vi "Fire Logging.vi"(11 "error in":errorcluster) -> ()   [LabVIEW 2015]
doc: "Converts an array of data to a row of tab-separated columns, prepends the timestamp column, and terminates each row with the end of line character."
uses:
  <vilib>/Rock Robotics/Network Tables/NT Read Number.vi
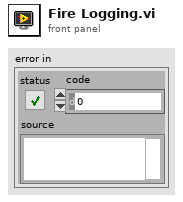
[diagram p1: front panel]
types:
  T1 = enum16{"open", "replace", "create", "open or create", "replace or create", "replace or create with confirmation"}
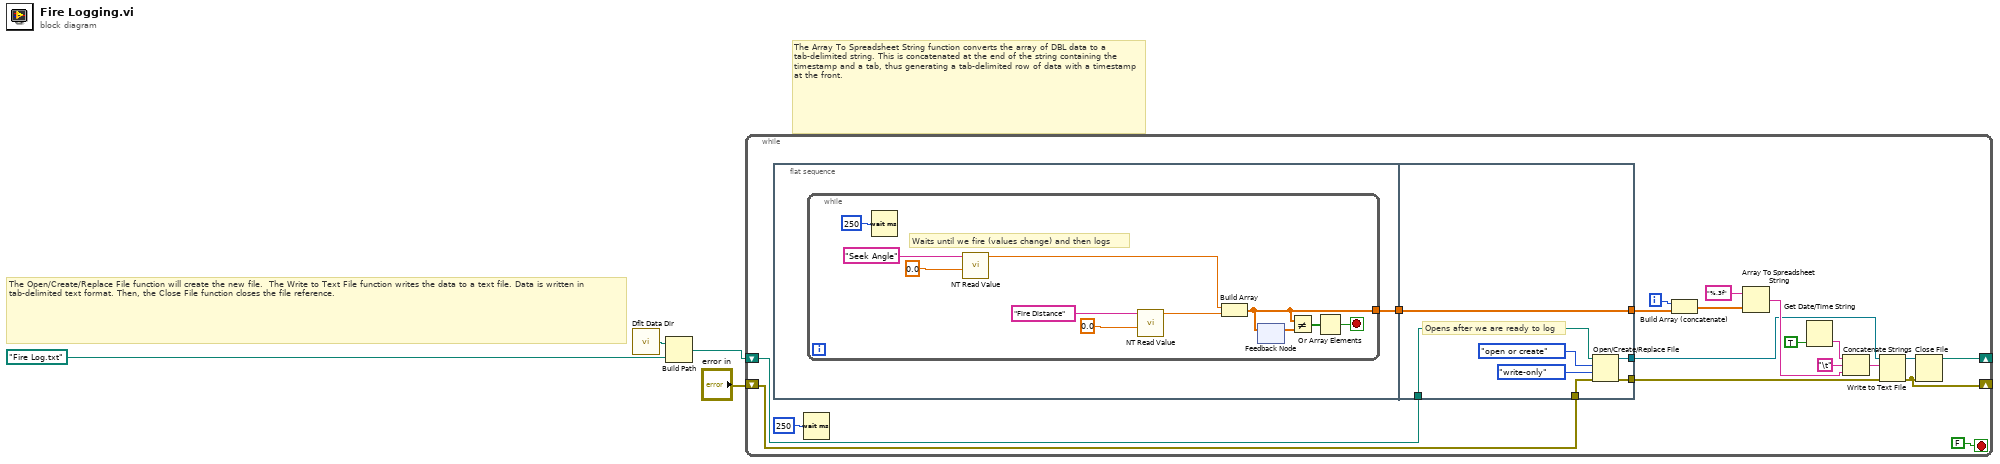
[diagram p0: block diagram]
diagram:
  # "The Array To Spreadsheet String function converts the array of DBL data to a tab-delimited string. This is concatenated at the end of the string containing the timestamp and a tab, thus generating a tab-delimited row of data with a timestamp at the front."
  # "The Open/Create/Replace File function will create the new file.  The Write to Text File function writes the data to a text file. Data is written in tab-delimited text format. Then, the Close File function closes the file reference."
  n1 = call <vilib>:"Dflt Data Dir.vi"() -> ("App:Default Data Directory"=w3:path)
  n2 = Build Path(base path=w3, name or relative path=path "Fire Log.txt" ("default name")) -> (appended path=w2:path)
  n3 = while {
    shift-right: [w13] -> _
    shift-left: w2 -> [w9]
    shift-right: [w15] -> _
    shift-left: "error in" -> [w10]
    i -> [w6]
    stop <- FALSE stop-if-true
    n4 = flat-sequence {
      tunnel: [w24] -> w12
      tunnel: [w42] -> w7
      tunnel: w12 -> [w42]
      tunnel: w9 -> [w39]
      tunnel: [w38] -> w11
      tunnel: w10 -> [w37]
      tunnel: [w36] -> w8
      frame #0 {
        n5 = while {
          tunnel: [w26] -> w24
          stop <- w27 stop-if-true
          # "Waits until we fire (values change) and then logs"
          n6 = Wait (ms)(milliseconds to wait=u32 250) -> ()  [unwired: 1 out]
          n7 = call-poly <vilib>:"NT Read Value.vi"("Default Value"=0.0, "Name"="Seek Angle") -> ("Numeric"=w31:dbl)  [unwired: 8 in, 1 out]
          n8 = call-poly <vilib>:"NT Read Value.vi"("Default Value"=0.0, "Name"="Fire Distance") -> ("Numeric"=w30:dbl)  [unwired: 8 in, 1 out]
          n9 = Build Array(w31, w30) -> (w26:dbl[])
          n10 = feedback-in #1(w26) -> ()
          n11 = feedback #1() -> (w29:dbl[])  [unwired: 1 in]
          n12 = Not Equal?(x=w26, y=w29) -> (x != y?=w28:bool[])
          n13 = Or Array Elements(Boolean array=w28) -> (logical OR=w27:bool)
        }
      }
      frame #1 {
        # "Opens after we are ready to log"
        n14 = Open/Create/Replace File(file path (use dialog)=w39, error in=w37, operation (0:open)=T1."open or create", access (0:read/write)=enum16{"read/write", "read-only", "write-only"}."write-only") -> (refnum out=w36:refnum<file>, error out=w38:errorcluster)  [unwired: 3 out]
      }
    }
    n15 = Wait (ms)(milliseconds to wait=u32 250) -> ()  [unwired: 1 out]
    n16 = Build Array (concatenate)(w6, w7) -> (w5:dbl[])
    n17 = Array To Spreadsheet String(array=w5, 3:"%.3f") -> (spreadsheet string=w22:string)  [unwired: 1 out]
    n18 = Get Date/Time String(want seconds? (F)=TRUE) -> (time string=w18:string)  [unwired: 2 in, 1 out]
    n19 = Concatenate Strings(w18, "\t" ("Tab"), w22) -> (w20:string)
    n20 = Write to Text File(file (use dialog)=w8, text=w20, error in=w11) -> (refnum out=w14:refnum<file>, error out=w15:errorcluster)  [unwired: 1 in, 1 out]
    n21 = Close File(refnum=w14, error in=w15) -> (path=w13:path)  [unwired: 1 out]
  }
